vi "lvpeak_get_frame.vi"(8 "error in (no error)":errorcluster, 10 "Image in":T1, 11 "camera_id":u64) -> (0 "error out":errorcluster, 2 "Image out":T1, 3 "camera_id out":u64)   [LabVIEW 2024, in "Vision.lvlib"]
uses:
  Vision.lvlib
  bin/LVPeak.dll
  <vilib>/vision/Image Controls.llb/IMAQ Image.ctl
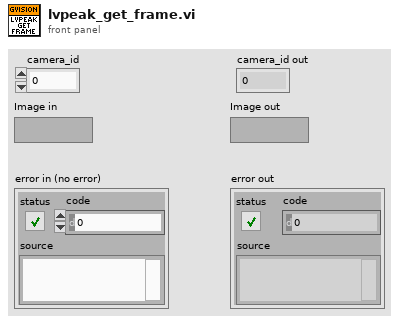
[diagram p1: front panel]
types:
  T1 = typedef "IMAQ Image.ctl" = refnum<image>
  T2 = enum32{"Map Pixel Pointer", "Unmap Pixel Pointer", "Get Pixels Infos"}
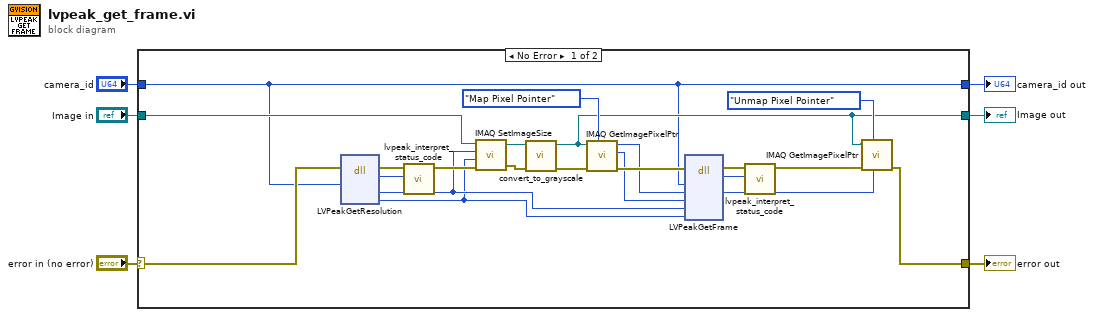
[diagram p0: block diagram]
diagram:
  n1 = case shown="No Error" "error in (no error)" {
    selector: "error in (no error)" -> [w24 w31]
    tunnel: [w9 w31] -> w5
    tunnel: "camera_id" -> [w7 w29]
    tunnel: "Image in" -> [w21 w30]
    tunnel: [w8 w30] -> w2
    tunnel: [w7 w29] -> w1
    frame No Error {
      n2 = dll-call lib="C:/Users/cfang/Desktop/nebraska-silicon-lab/pixel-gantry-control/Gantry/Shared Components/bin/LVPeak.dll" fn="LVPeakGetResolution"(error in=w24, "camera_id"=w7) -> (error out=w28:errorcluster, "return type"=w27:i32, "width_px"=w15:u32, "height_px"=w14:u32)  [unwired: 5 in, 1 out]
      n3 = call "lvpeak_interpret_status_code.vi"("status_code"=w27, "error in (no error)"=w28) -> ("error out"=w22:errorcluster)  [unwired: 9 in]
      n4 = call "IMAQ SetImageSize"("error in (no error)"=w22, "Y Resolution"=w14, "X Resolution"=w15, "Image"=w21) -> ("error out"=w19:errorcluster, "Image Out"=w20:T1)  [unwired: 1 in]
      n5 = call "convert_to_grayscale.vi"("error in (no error)"=w19, "Image in"=w20) -> ("error out"=w18:errorcluster, "Image out"=w8:T1)  [unwired: 8 in]
      n6 = call "IMAQ GetImagePixelPtr"("Function"=T2."Map Pixel Pointer", "error in (no error)"=w18, "Image"=w8) -> ("error out"=w17:errorcluster, "LineWidth(Pixels)"=w16:i32, "Pixel Pointer out"=w12:u64)  [unwired: 3 in, 3 out]
      n7 = dll-call lib="C:/Users/cfang/Desktop/nebraska-silicon-lab/pixel-gantry-control/Gantry/Shared Components/bin/LVPeak.dll" fn="LVPeakGetFrame"(error in=w17, "camera_id"=w7, "imgPtr"=w12, "imgLineWidth"=w16, "imgWidth"=w15, "imgHeight"=w14) -> (error out=w26:errorcluster, "return type"=w25:i32, "imgPtr"=w11:u64)  [unwired: 6 in, 1 out]
      n8 = call "lvpeak_interpret_status_code.vi"("status_code"=w25, "error in (no error)"=w26) -> ("error out"=w13:errorcluster)  [unwired: 9 in]
      n9 = call "IMAQ GetImagePixelPtr"("Pixel Pointer in"=w11, "Function"=T2."Unmap Pixel Pointer", "error in (no error)"=w13, "Image"=w8) -> ("error out"=w9:errorcluster)  [unwired: 2 in, 5 out]
    }
    frame Error {
    }
  }
  "error out" <- w5
  "Image out" <- w2
  "camera_id out" <- w1
